vi "Read SEQ.vi"(8 "error in":errorcluster, 10 "Created New?":bool, 11 "Local Instance Event SEQ":refnum<queue>) -> (0 "error out":errorcluster, 3 "Local Instance Request Events":T1)   [LabVIEW 2024, in "CTIWrapper.lvlib" / "Local Instance Events SEQ.lvlib"]
doc: "_____\nCreated using DQMH Framework: Event Scripter 7.1.0.1503."
uses:
  Local Instance Events SEQ.lvlib
  Local Instance Request Events--cluster.ctl
  Wake Up CT HL Argument--cluster.ctl
  CTIWrapper.lvlib
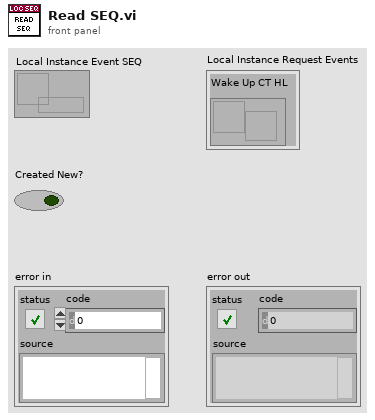
[diagram p1: front panel]
types:
  T1 = typedef "CTIWrapper.lvlib/Local Instance Request Events--cluster.ctl" = cluster{"Wake Up CT HL":refnum<user-event>}
  T2 = typedef "CTIWrapper.lvlib/Wake Up CT HL Argument--cluster.ctl" = cluster{"Module ID":i32, "VISA resource name":refnum<visa-resource-name>}
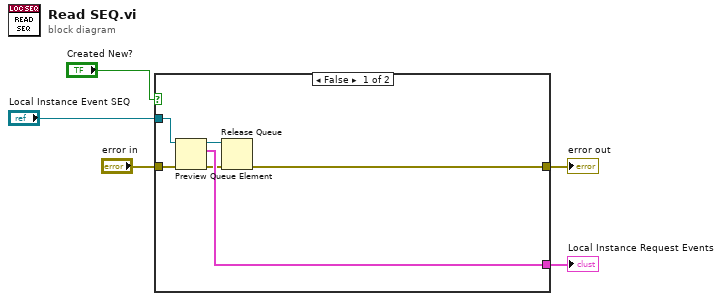
[diagram p0: block diagram]
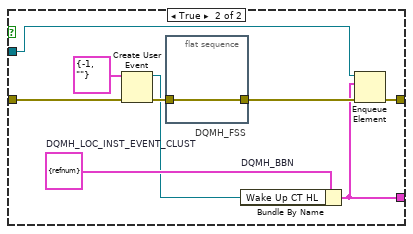
[diagram p2: hidden frame]
diagram:
  n1 = case shown="False" "Created New?" {
    tunnel: "error in" -> [w11 w19]
    tunnel: [w7 w20] -> w4
    tunnel: [w10 w15] -> w2
    tunnel: "Local Instance Event SEQ" -> [w9 w17]
    frame False {
      n2 = Preview Queue Element(queue=w9, error in (no error)=w11) -> (queue out=w6:refnum<queue>, element=w10:T1, error out=w8:errorcluster)  [unwired: 1 in, 1 out]
      n3 = Release Queue(queue=w6, error in (no error)=w8) -> (error out=w7:errorcluster)  [unwired: 1 in, 2 out]
    }
    frame True {
      w16 = T1 {"Wake Up CT HL"=refnum}  # DQMH_LOC_INST_EVENT_CLUST
      n4 = Create User Event(user event datatype=T2 {"Module ID"=-1, "VISA resource name"=""} ("Wake Up CT HL Argument"), error in=w19) -> (user event=w12:refnum<user-event>, error out=w14:errorcluster)
      n5 = flat-sequence "DQMH_FSS" {
        tunnel: w14 -> [w21]
        tunnel: [w21] -> w18
        frame #0 {
        }
      }
      n6 = Bundle By Name "DQMH_BBN"(cluster=w16, "Wake Up CT HL"=w12) -> (w15:T1)
      n7 = Enqueue Element(queue=w17, element=w15, error in (no error)=w18) -> (error out=w20:errorcluster)  [unwired: 1 in, 2 out]
    }
  }
  "error out" <- w4
  "Local Instance Request Events" <- w2
